vi "Get XML file path.vi"(8 "Error In":errorcluster, 10 "Class name":string, 11 "Application Name":string) -> (0 "Error Out":errorcluster, 2 "File exists?":bool, 3 "Path for XML file":path)   [LabVIEW 2020, in "Test Framework.lvclass"]
doc: "Gets the XML file path for a given application and class name.\nIt uses the users location for AppData from Registration database.\nThis enables multiple users to have different settings for the same application"
uses:
  Test Framework.lvclass
  <vilib>/registry/registry.llb/Registry RtKey.ctl
  <vilib>/registry/registry.llb/Read Registry Value Simple STR.vi
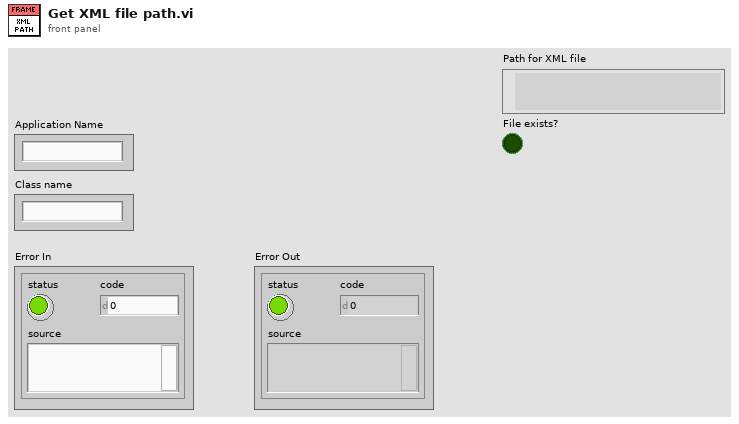
[diagram p1: front panel]
types:
  T1 = typedef "Registry RtKey.ctl" = enum32{"HKEY_CLASSES_ROOT", "HKEY_CURRENT_USER", "HKEY_LOCAL_MACHINE", "HKEY_USERS", "HKEY_PERFORMANCE_DATA", "HKEY_CURRENT_CONFIG", "HKEY_DYN_DATA"}
  T2 = typedef "Registry refnum.ctl" = refnum<k1>
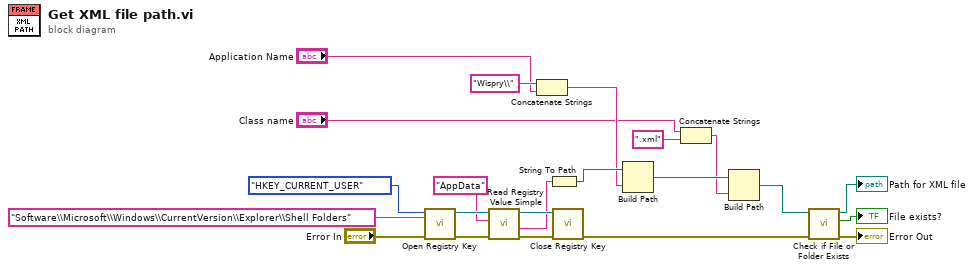
[diagram p0: block diagram]
diagram:
  n1 = call <vilib>:"Open Registry Key.vi"("error in (no error)"="Error In", "subkey"="Software\\Microsoft\\Windows\\CurrentVersion\\Explorer\\Shell Folders", "root key (HKEY_LOCAL_MACHINE)"=Registry_RtKey."HKEY_CURRENT_USER") -> ("error out"=w20:errorcluster, "refnum out"=w19:T2)  [unwired: 7 in]
  n2 = call-poly <vilib>:"Read Registry Value Simple.vi"("error in (no error)"=w20, "value"="AppData", "refnum"=w19) -> ("error out"=w17:errorcluster, "String/Binary data"=w12:string, "refnum out"=w16:T2)  [unwired: 3 in, 1 out]
  n3 = Concatenate Strings("Wispry\\" ("string"), "Application Name") -> (w10:string)
  n4 = String To Path(string=w12) -> (path=w11:path)
  n5 = call <vilib>:"Close Registry Key.vi"("error in (no error)"=w17, "refnum"=w16) -> ("error out"=w4:errorcluster)  [unwired: 5 in]
  n6 = Build Path(base path=w11, name or relative path=w10) -> (appended path=w7:path)
  n7 = Concatenate Strings("Class name", ".xml" ("string")) -> (w6:string)
  n8 = Build Path(base path=w7, name or relative path=w6) -> (appended path=w5:path)
  n9 = call <vilib>:"Check if File or Folder Exists.vi"("error in (no error)"=w4, "path"=w5) -> ("error out"=→"Error Out":errorcluster, "file or folder exists?"=→"File exists?":bool, "dup path"=→"Path for XML file":path)  [unwired: 7 in]
